vi "StepsInit.vi"(8 "Feedback":T2, 9 "Auto":bool, 10 "Inicjalizuj":bool) -> (3 "Cluster":T3)   [LabVIEW 2020]
uses:
  controls/Data.ctl
panel:
  in  "error":errorcluster
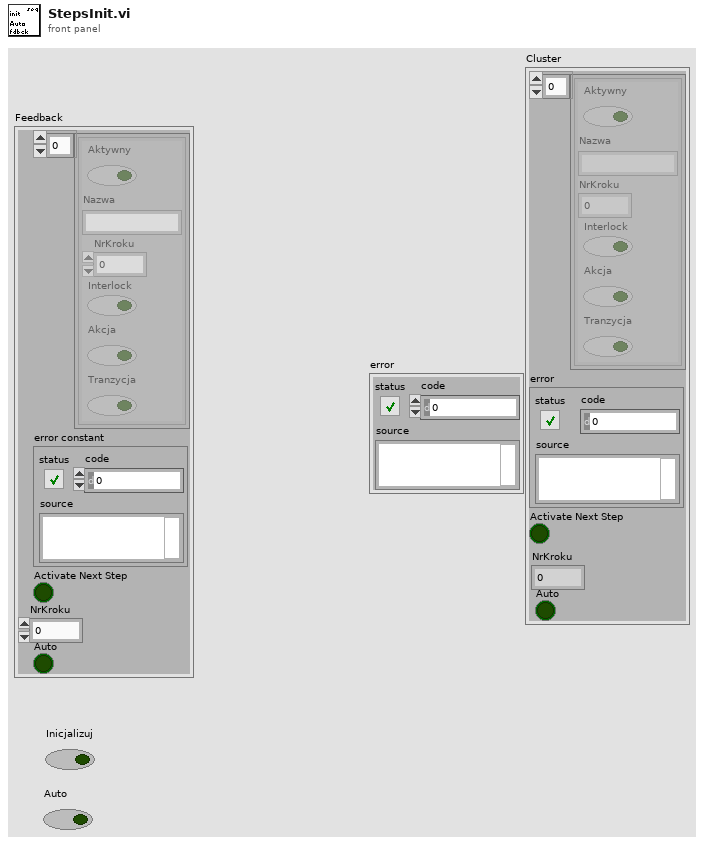
[diagram p1: front panel]
types:
  T1 = typedef "Data.ctl" = cluster{"Aktywny":bool, "Nazwa":string, "NrKroku":dbl, "Interlock":bool, "Akcja":bool, "Tranzycja":bool}
  T2 = cluster{T1[], "error constant":errorcluster, "Activate Next Step":bool, "NrKroku":dbl, "Auto":bool}
  T3 = cluster{T1[], "error":errorcluster, "Activate Next Step":bool, "NrKroku":dbl, "Auto":bool}
  T4 = cluster{T1[], "error":errorcluster, "Boolean <Replace Me>":bool, i32, "Auto":bool}
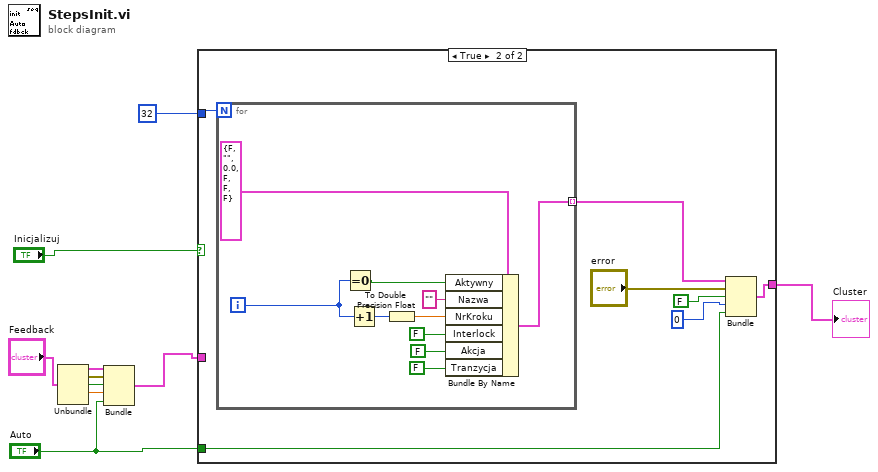
[diagram p0: block diagram]
diagram:
  n1 = Unbundle("Feedback") -> (w3:T1[], "error constant"=w4:errorcluster, "Activate Next Step"=w5:bool, "NrKroku"=w6:dbl)  [unwired: 1 out]
  n2 = Bundle(w3, "error constant"=w4, "Activate Next Step"=w5, "NrKroku"=w6, "Auto"="Auto") -> (w2:T2)  [unwired: 1 in]
  n3 = case shown="True" "Inicjalizuj" {
    tunnel: 32 ("MaxStep") -> [_ w18]
    tunnel: [w11 w13] -> w9
    tunnel: w2 -> [w11 _]
    tunnel: "Auto" -> [_ w12]
    frame False {
    }
    frame True {
      n4 = for {
        N: w18 -> [_]
        tunnel: [w27] -> w17 mode=indexing
        i -> [w22]
        n5 = Equal To 0?(x=w22) -> (x = 0?=w21:bool)
        n6 = Increment(x=w22) -> (x+1=w20:i32)
        n7 = To Double Precision Float(number=w20) -> (double precision float=w19:dbl)
        n8 = Bundle By Name(cluster=T1 {"Aktywny"=FALSE, "Nazwa"="", "NrKroku"=0.0, "Interlock"=FALSE, "Akcja"=FALSE, "Tranzycja"=FALSE} ("Krok 2"), "Aktywny"=w21, "Nazwa"="", "NrKroku"=w19, "Interlock"=FALSE ("Boolean <Replace Me>"), "Akcja"=FALSE ("Boolean <Replace Me>"), "Tranzycja"=FALSE ("Boolean <Replace Me>")) -> (w27:T1)
      }
      n9 = Bundle(w17, "error"="error", "Boolean <Replace Me>"=FALSE, 0, "Auto"=w12) -> (w13:T4)  [unwired: 1 in]
    }
  }
  "Cluster" <- w9
